vi "Configure SRL Measurement.vi"(5 "Manual Impedance Value (50 ohm)":dbl=50.0, 6 "Cutoff Frequency (2.1E+8)":dbl=210000000.0, 7 "Enable Auto Impedance (T: Enable)":bool=TRUE, 8 "error in (no error)":errorcluster, 9 "Enable SRL (F: Disable)":bool, 10 "Channel (1)":i32=1, 11 "VISA resource name":refnum<visa-resource-name>) -> (0 "error out":errorcluster, 3 "VISA resource name out":refnum<visa-resource-name>)   [LabVIEW 2011, in "Agilent ENA Series.lvlib"]
doc: "This VI configures SRL measurement.\n\n<B>Note:</B>This VI is only vaild on E5061B."
uses:
  Agilent ENA Series.lvlib
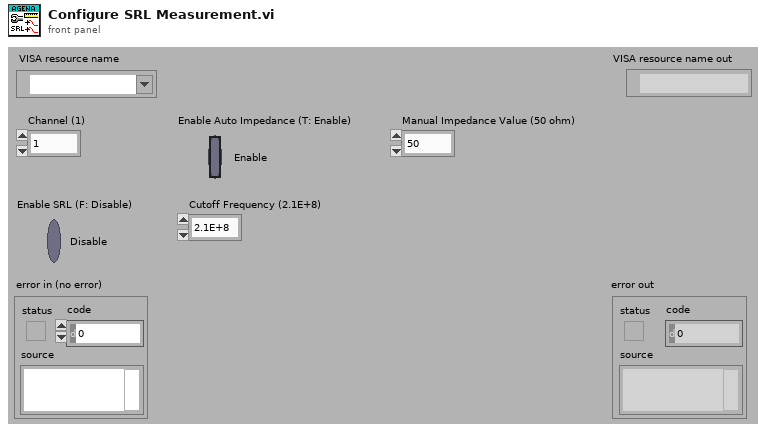
[diagram p1: front panel]
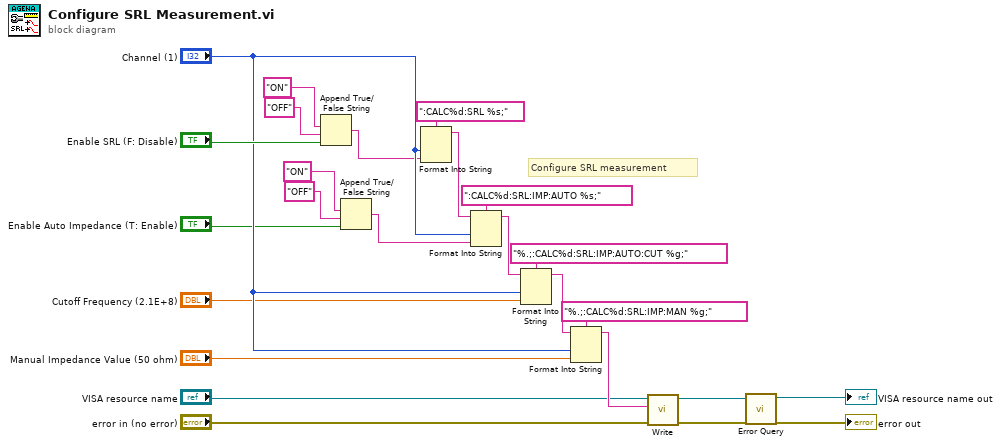
[diagram p0: block diagram]
diagram:
  # "Configure SRL measurement"
  n1 = Append True/False String(1:"Enable SRL (F: Disable)", 2:"OFF", 3:"ON") -> (0:w20:string)  [unwired: 1 out]
  n2 = Append True/False String(1:"Enable Auto Impedance (T: Enable)", 2:"OFF", 3:"ON") -> (0:w15:string)  [unwired: 1 out]
  n3 = Format Into String(format string=":CALC%d:SRL %s;", "Channel (1)", w20) -> (resulting string=w8:string)  [unwired: 2 in, 1 out]
  n4 = Format Into String(format string=":CALC%d:SRL:IMP:AUTO %s;", initial string=w8, "Channel (1)", w15) -> (resulting string=w7:string)  [unwired: 1 in, 1 out]
  n5 = Format Into String(format string="%.;:CALC%d:SRL:IMP:AUTO:CUT %g;", initial string=w7, "Channel (1)", "Cutoff Frequency (2.1E+8)") -> (resulting string=w6:string)  [unwired: 1 in, 1 out]
  n6 = Format Into String(format string="%.;:CALC%d:SRL:IMP:MAN %g;", initial string=w6, "Channel (1)", "Manual Impedance Value (50 ohm)") -> (resulting string=w5:string)  [unwired: 1 in, 1 out]
  n7 = call "Write.vi"("error in (no error)"="error in (no error)", "String ()"=w5, "VISA resource name"="VISA resource name") -> ("error out"=w1:errorcluster, "VISA resource name out"=w2:refnum<visa-resource-name>)  [unwired: 6 in, 1 out]
  n8 = call "Error Query.vi"("error in (no error)"=w1, "VISA resource name"=w2) -> ("error out"=→"error out":errorcluster, "VISA resource name out"=→"VISA resource name out":refnum<visa-resource-name>)  [unwired: 8 out]
